vi "onHarvestPips.vi"(7 "Environment in":refnum<class "Environment.lvclass">, 11 "Pips":refnum<class "Pips.lvclass">) -> (0 "error out":errorcluster, 3 "Pips":refnum<class "Pips.lvclass">)   [LabVIEW 2021, in "Bananas.lvlib" / "Environment.lvclass"]
uses:
  Environment.lvclass
  Pips/Pips.lvclass
  BananaPeel/BananaPeel.lvclass
  Environment.lvclass/Environment.ctl
  <vilib>/LabVIEW Open Source Project/Cryptographic Functions/SHA-1/SHA-1.vi
  <vilib>/LabVIEW Open Source Project/Data Manipulation/Variant/Variant_EmptyCluster.vi
  <vilib>/LabVIEW Open Source Project/Data Manipulation/TypeDescriptor/TypeDescriptor_SetName.vi
  <vilib>/Utility/GetType.llb/TD_Create Cluster.vi
  <vilib>/LabVIEW Open Source Project/Cryptographic Functions/SHA-1/SHA-1.lvclass
  <vilib>/LabVIEW Open Source Project/Data Manipulation/Variant/OpenVariant.lvlib
  <vilib>/LabVIEW Open Source Project/Cryptographic Functions/SHA-1/SHA-1.lvlib
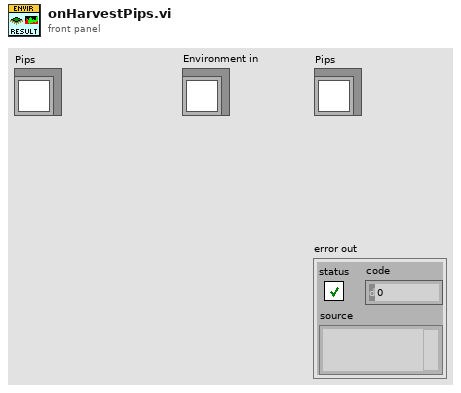
[diagram p1: front panel]
types:
  T1 = enum32{"invalid app kind", "Development System", "Run Time System", "Student Edition", "Embedded LabVIEW", "Evaluation", "Custom"}
  T2 = cluster{"Timestamp.ConfiguredAt":string, "Timestamp.UTCOffset":string, "Timestamp.Unix":string, "OS.DetailedName":string, "OS.Name":string, "OS.Version":string, "OS.BuildNumber":string, "App.Language":string, "App.Kind":string, "App.Language":string, "App.VersionYear":string, "App.Version":string, "App.Name":string}
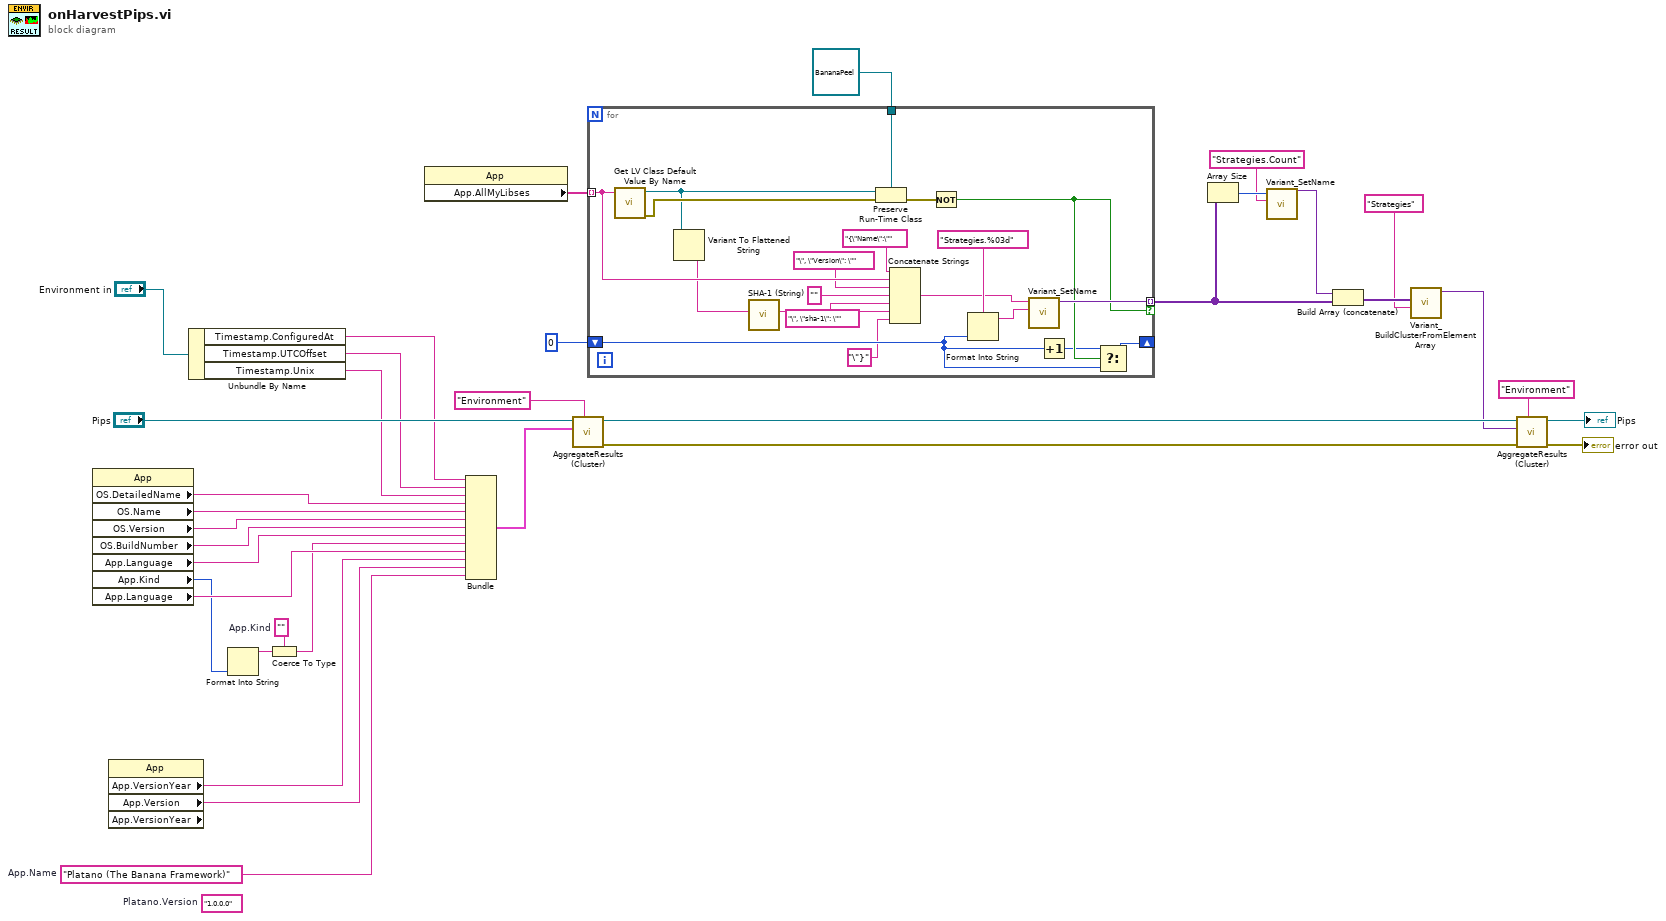
[diagram p0: block diagram]
diagram:
  (unwired) "1.0.0.0"  # Platano.Version
  w20 = "Platano (The Banana Framework)"  # App.Name
  w25 = ""  # App.Kind
  n1 = property class="App"() -> ("OS.DetailedName"=w34:string, "OS.Name"=w33:string, "OS.Version"=w32:string, "OS.BuildNumber"=w27:string, "App.Language"=w30:string, "App.Kind"=w24:T1, "App.Language"=w28:string)  [unwired: 2 in, 2 out]
  n2 = property class="App" props=["App.VersionYear", "App.Version", "App.VersionYear"]() -> ("App.VersionYear"=w22:string, "App.Version"=w21:string)  [unwired: 2 in, 3 out]
  n3 = Unbundle By Name("Environment in") -> ("Timestamp.ConfiguredAt"=w19:string, "Timestamp.UTCOffset"=w18:string, "Timestamp.Unix"=w17:string)
  n4 = Format Into String(w24) -> (resulting string=w26:string)  [unwired: 3 in, 1 out]
  n5 = Coerce To Type(0:w26, 1:w25) -> (2:w23:string)
  n6 = property class="App"() -> ("App.AllMyLibses"=w11:string[])  [unwired: 2 in, 2 out]
  n7 = Bundle("Timestamp.ConfiguredAt"=w19, "Timestamp.UTCOffset"=w18, "Timestamp.Unix"=w17, "OS.DetailedName"=w34, "OS.Name"=w33, "OS.Version"=w32, "OS.BuildNumber"=w27, "App.Language"=w30, "App.Kind"=w23, "App.Language"=w28, "App.VersionYear"=w22, "App.Version"=w21, "App.Name"=w20) -> (w31:T2)  [unwired: 1 in]
  n8 = call "AggregateResults (Cluster).vi"("Section"="Environment", "Value"=w31, "Pips in"="Pips") -> ("error out"=w14:errorcluster, "Pips out"=w16:refnum<class "Pips.lvclass">)  [unwired: 7 in]
  n9 = for {
    tunnel: w11 -> [w45] mode=indexing
    tunnel: refnum<class "BananaPeel.lvclass"> refnum ("Bananas.lvlib:BananaPeel.lvclass") -> [w55]
    tunnel: [w50] -> w3 mode=indexing if=w48
    shift-right: [w49] -> _
    shift-left: 0 -> [w46]
    n10 = call <vilib>:"Get LV Class Default Value By Name.vi"("class name"=w45) -> ("error out"=w54:errorcluster, "object"=w37:refnum<class>)  [unwired: 9 in]
    n11 = Variant To Flattened String(Variant=w37) -> (data string=w36:string)  [unwired: 1 out]
    n12 = call <vilib>:"SHA-1 (String).vi"("message"=w36) -> ("SHA-1 hash"=w39:string)  [unwired: 10 in]
    n13 = Preserve Run-Time Class(object in=w37, error in=w54, 2:w55) -> (error out=w53:errorcluster)  [unwired: 1 out]
    n14 = Concatenate Strings("{\"Name\":\"" ("string"), w45, "\", \"Version\": \"" ("string"), "" ("string"), "\", \"sha-1\": \"" ("string"), w39, "\"}" ("string")) -> (w44:string)
    n15 = Not(x=w53) -> (.not. x?=w48:bool)
    n16 = Format Into String(format string="Strategies.%03d", w46) -> (resulting string=w52:string)  [unwired: 2 in, 1 out]
    n17 = call <vilib>:"Variant_SetName.vi"("Name"=w52, "Variant"=w44) -> ("Named Variant"=w50:variant)  [unwired: 9 in]
    n18 = Increment(x=w46) -> (x+1=w47:i32)
    n19 = Select(t=w47, s=w48, f=w46) -> (s? t:f=w49:i32)
  }
  n20 = Array Size(array=w3) -> (size(s)=w8:i32)
  n21 = call <vilib>:"Variant_SetName.vi"("Name"="Strategies.Count", "Variant"=w8) -> ("Named Variant"=w7:variant)  [unwired: 9 in]
  n22 = Build Array (concatenate)(w7, w3) -> (w6:variant[])
  n23 = call <vilib>:"Variant_BuildClusterFromElementArray.vi"("name"="Strategies", "Elements"=w6) -> ("Cluster"=w4:variant)  [unwired: 9 in]
  n24 = call "AggregateResults (Cluster).vi"("Section"="Environment", "error in (no error)"=w14, "Value"=w4, "Pips in"=w16) -> ("error out"=→"error out":errorcluster, "Pips out"=→"Pips":refnum<class "Pips.lvclass">)  [unwired: 6 in]
